vi "Do.vi"(8 "error in (no error)":errorcluster, 10 "Actor in":refnum<class "Actor.lvclass">, 11 "3_UpdateSubscribeList Msg in":refnum<class "3_UpdateSubscribeList Msg.lvclass">) -> (0 "error out":errorcluster, 2 "Actor out":refnum<class "Actor.lvclass">)   [LabVIEW 2018, in "MQTT_Client_Actor.lvlib" / "3_UpdateSubscribeList Msg.lvclass"]
doc: "(<B>Filename</B>: Actor Framework.lvlib:Message.lvclass:Do.vi)\n\nDefines what a message does when it is received by an actor. Generally, a message instructs an actor to invoke one of its methods. By default, this method does nothing. A child class must override it to define behavior. Create a child class by using the Actor Framework Message Maker dialog box."
uses:
  3_UpdateSubscribeList Msg.lvclass
  <vilib>/ActorFramework/Actor/Actor.lvclass
  MQTT_Client_Actor/MQTT_Client_Actor.lvclass
  D:/Program Files (x86)/National Instruments/LabVIEW 2018/vi.lib/ActorFramework/Actor/Actor.lvclass
  3_UpdateSubscribeList Msg.lvclass/3_UpdateSubscribeList Msg.ctl
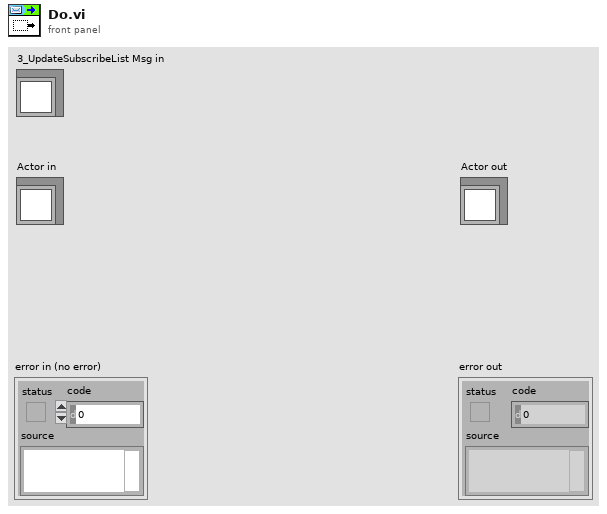
[diagram p1: front panel]
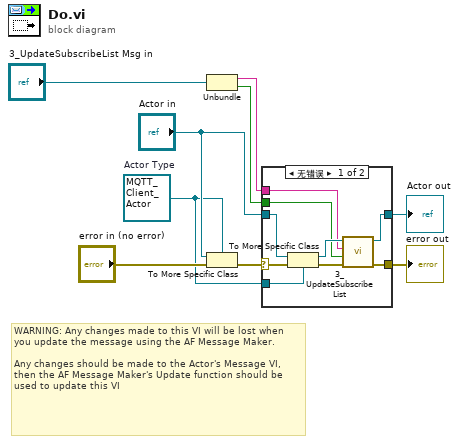
[diagram p0: block diagram]
diagram:
  w4 = refnum<class "MQTT_Client_Actor.lvclass"> refnum  # Actor Type
  # "WARNING: Any changes made to this VI will be lost when you update the message using the AF Message Maker.\n\nAny changes should be made to the Actor's Message VI, then the AF Message Maker's Update function should be used to update this VI"
  n1 = Unbundle("3_UpdateSubscribeList Msg in") -> (w3:string, w2:bool)
  n2 = To More Specific Class ("转换为特定的类")(target class=w4, reference="Actor in", error in="error in (no error)") -> (error out=w8:errorcluster)  [unwired: 1 out]
  n3 = case shown="无错误" w8 {
    selector: w8 -> [w18 w20]
    tunnel: [w10 w20] -> w7
    tunnel: [w11 w19] -> w6
    tunnel: "Actor in" -> [w17 w19]
    tunnel: w4 -> [w16 _]
    tunnel: w3 -> [w13 _]
    tunnel: w2 -> [w12 _]
    frame No Error {
      n4 = To More Specific Class ("Actor Cast")(target class=w16, reference=w17, error in=w18) -> (specific class reference=w15:refnum<class "MQTT_Client_Actor.lvclass">, error out=w14:errorcluster)
      n5 = call "3_UpdateSubscribeList.vi"("error in (no error)"=w14, "T:Add"=w12, "Topic"=w13, "MQTT_Client_Actor 输入"=w15) -> ("error out"=w10:errorcluster, "MQTT_Client_Actor 输出"=w11:refnum<class "MQTT_Client_Actor.lvclass">)  [unwired: 6 in]
    }
    frame Error {
    }
  }
  "error out" <- w7
  "Actor out" <- w6
